vi "My OFDM RX.vi"() -> ()   [LabVIEW 2013]
uses:
  <vilib>/Analysis/2dsp.llb/Complex FFT.vi
  <vilib>/addons/Modulation/Digital/General/MT Map QAM Symbols to Bits.vi
  <vilib>/addons/Modulation/niAMT.lvlib
  <vilib>/Analysis/NI_AALPro.lvlib
  <vilib>/addons/Modulation/niDMT.lvlib
panel:
  out "Constellation":cdb[](graph)
  out "Complex baseband":cluster{"t0":dbl, "dt":dbl, "Y":dbl[]}[](graph)
  out "output cluster":cluster{bool[], bool[]}
  in  "stop":bool
  in  "desired sample rate (Hz)":dbl=1.0 format="%.2f"
  out "error out":errorcluster
  out "Bit Error":dbl
  in  "error in (no error)":errorcluster
  in  "queue size":i32
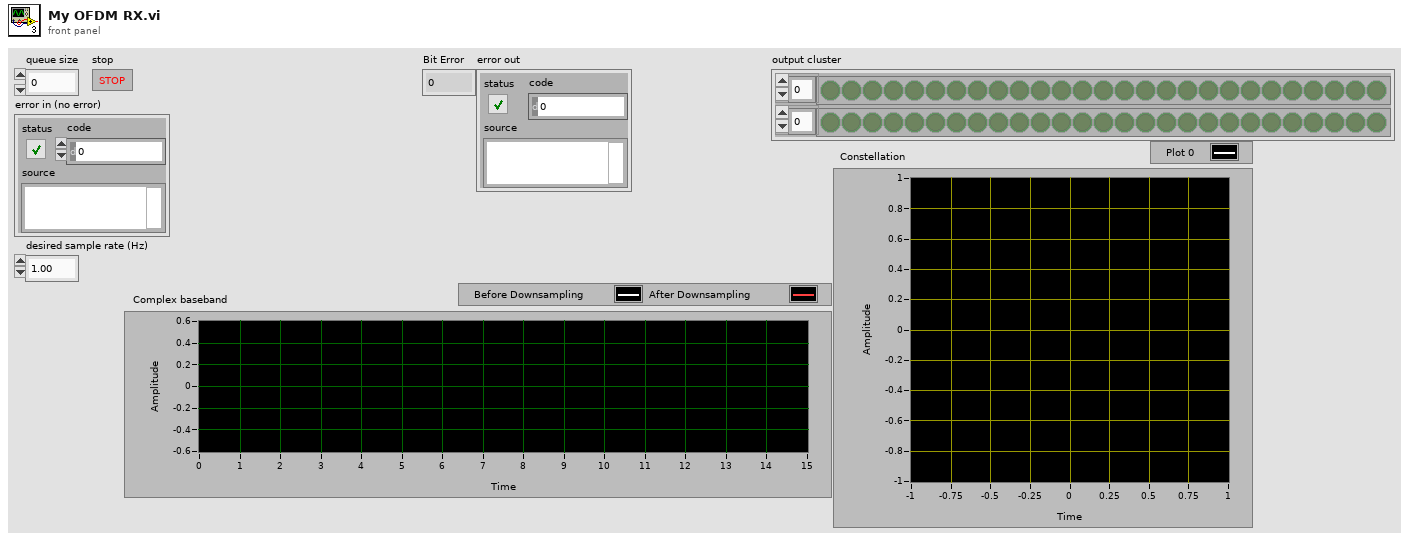
[diagram p1: front panel]
types:
  T1 = cluster{"IQ Data":cdb[], "Original Bitstream":i8[]}
  T2 = typedef "niAMT.lvlib/Complex Data Waveform.ctl" = cluster{"t0":dbl, "dt":dbl, "Y":cdb[]}
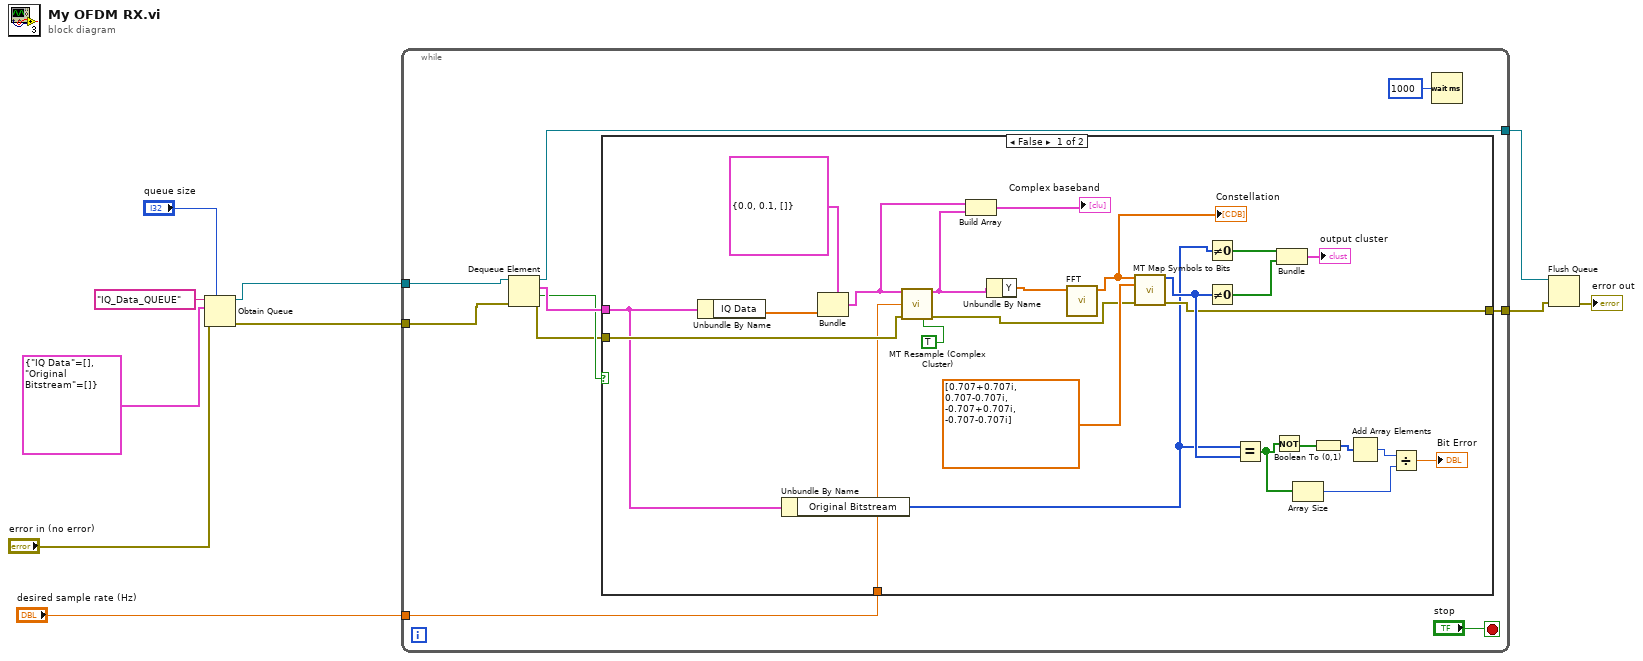
[diagram p0: block diagram]
diagram:
  n1 = Obtain Queue(max queue size (-1, unlimited)="queue size", name (unnamed)="IQ_Data_QUEUE", element data type=T1 {"IQ Data"=[], "Original Bitstream"=[]}, error in (no error)="error in (no error)") -> (queue out=w8:refnum<queue>, error out=w6:errorcluster)  [unwired: 1 in, 1 out]
  n2 = while {
    tunnel: w8 -> [w20]
    tunnel: w6 -> [w19]
    tunnel: [w15] -> w5
    tunnel: "desired sample rate (Hz)" -> [w14]
    tunnel: [w13] -> w2
    stop <- "stop" stop-if-true
    n3 = Dequeue Element(queue=w20, error in (no error)=w19) -> (queue out=w13:refnum<queue>, element=w18:T1, timed out?=w17:bool, error out=w16:errorcluster)  [unwired: 1 in]
    n4 = case shown="False" w17 {
      tunnel: w18 -> [w36 _]
      tunnel: w16 -> [w44 w46]
      tunnel: [w27 w46] -> w15
      tunnel: w14 -> [w26 _]
      frame False {
        n5 = Unbundle By Name(w36) -> ("IQ Data"=w25:cdb[])
        n6 = Unbundle By Name(w36) -> ("Original Bitstream"=w24:i8[])
        n7 = Bundle(cluster=cluster{dbl, dbl, cdb[]} {0.0, 0.1, []}, w25) -> (w43:cluster{dbl, dbl, cdb[]})  [unwired: 2 in]
        n8 = call <vilib>:"MT Resample (Complex Cluster).vi"("input complex waveform"=w43, "desired sample rate (Hz)"=w26, "error in (no error)"=w44, "flush buffers? (F)"=TRUE) -> ("output complex waveform"=w42:T2, "error out"=w28:errorcluster)  [unwired: 10 in]
        n9 = Build Array(w43, w42) -> (→"Complex baseband":T2[])
        n10 = Unbundle By Name(w42) -> ("Y"=w40:cdb[])
        n11 = call-poly <vilib>:"FFT.vi"("X"=w40) -> ("FFT {X}"=w21:cdb[])  [unwired: 9 in, 1 out]
        "Constellation" <- w21
        n12 = call-poly <vilib>:"MT Map Symbols to Bits.vi"("symbols"=w21, "symbol map"=cdb[] [0.707+0.707i, 0.707-0.707i, -0.707+0.707i, -0.707-0.707i], "error in (no error)"=w28) -> ("output bit stream"=w35:i8[], "error out"=w27:errorcluster)  [unwired: 11 in]
        n13 = Not Equal To 0?(x=w24) -> (x != 0?=w38:bool[])
        n14 = Not Equal To 0?(x=w35) -> (x != 0?=w37:bool[])
        n15 = Equal?(x=w24, y=w35) -> (x = y?=w31:bool[])
        n16 = Not(x=w31) -> (.not. x?=w34:bool[])
        n17 = Bundle(w38, w37) -> (→"output cluster":cluster{bool[], bool[]})  [unwired: 1 in]
        n18 = Array Size(array=w31) -> (size(s)=w30:i32)
        n19 = Boolean To (0,1)(Boolean=w34) -> (0, 1=w33:i16[])
        n20 = Add Array Elements(numeric array=w33) -> (sum=w32:i16)
        n21 = Divide(x=w32, y=w30) -> (x/y=→"Bit Error":dbl)
      }
      frame True {
      }
    }
    n22 = Wait (ms)(milliseconds to wait=u32 1000) -> ()  [unwired: 1 out]
  }
  n23 = Flush Queue(queue=w2, error in (no error)=w5) -> (error out=→"error out":errorcluster)  [unwired: 2 out]
